vi "GL_BrkPtPRF.vi"(0 "GL Ref Out":refnum<k7>, 1 "Program Name":string caption="Beginning Text", 2 "PRF (1 ms)":u32=1 min=1 max=2147483647, 3 "error in":errorcluster) -> (5 "ref out":refnum<k7>, 7 "error out":errorcluster)   [LabVIEW 2022 SP3]
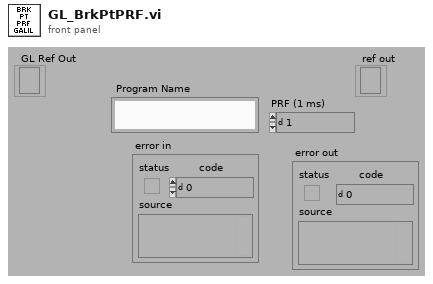
[diagram p1: front panel]
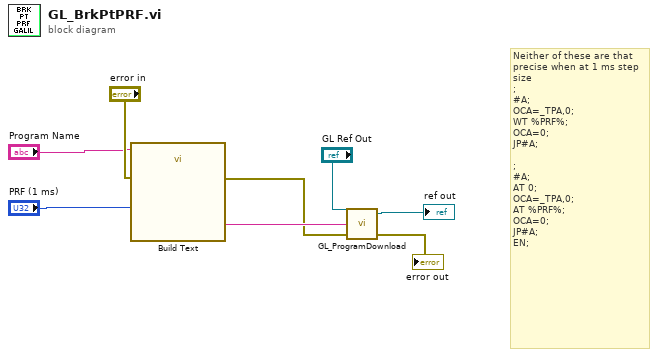
[diagram p0: block diagram]
diagram:
  # "Neither of these are that precise when at 1 ms step size\n;\n#A;\nOCA=_TPA,0;\nWT %PRF%;\nOCA=0;\nJP#A;\n\n;\n#A;\nAT 0;\nOCA=_TPA,0;\nAT %PRF%;\nOCA=0;\nJP#A;\nEN;"
  n1 = call "Build Text"("Beginning Text"="Program Name", "PRF"="PRF (1 ms)", "error in (no error)"="error in") -> ("Result"=w5:string, "error out"=w2:errorcluster)  [unwired: 11 in]
  n2 = call "GL_ProgramDownload.vi"("error in"=w2, "program"=w5, "Galil.IGalil"="GL Ref Out") -> ("error out"=→"error out":errorcluster, "reference out"=→"ref out":refnum<k7>)  [unwired: 1 out]
